vi "StdErr.vi"(11 "2D Array":u64[][](array[numeric]) format="%.1f") -> (0 "Deviation by row":i64[][](array[numeric]) format="%.1f", 1 "STD":dbl[](array[numeric]) format="%#_3g", 2 "Variance":dbl[](array[numeric]) format="%#_4g", 3 "Average by row":u64[](array[numeric]) format="%-2.1f", 4 "Mean as number":dbl format="%#_3g")   [LabVIEW 2023]
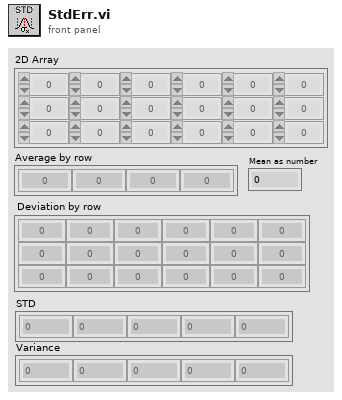
[diagram p1: front panel]
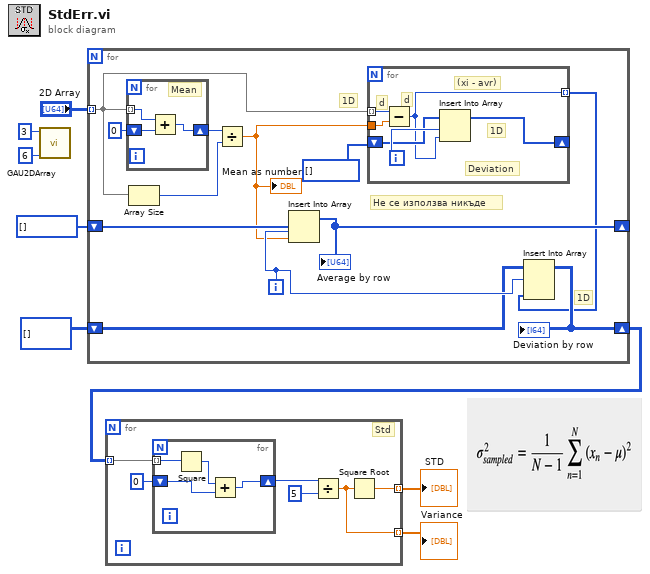
[diagram p0: block diagram]
diagram:
  n1 = call "GAU2DArray.vi"("Colums"=6, "Rows"=3) -> ()  [unwired: 8 in, 2 out]
  n2 = for {
    tunnel: "2D Array" -> [w11] mode=indexing
    shift-right: [w16] -> _
    shift-left: u64[] [] -> [w19]
    shift-right: [w13] -> w3
    shift-left: i64[][] [] -> [w14]
    i -> [w15]
    # "Не се използва никъде"
    # "1D"
    # "1D"
    n3 = for {
      tunnel: w11 -> [w29] mode=indexing
      shift-right: [w28] -> w18
      shift-left: 0 -> [w27]
      # "Mean"
      n4 = Add(x=w29, y=w27) -> (x+y=w28:u64)
    }
    n5 = Array Size(array=w11) -> (size(s)=w9:i32)
    n6 = Divide(x=w18, y=w9) -> (x/y=w12:dbl)
    "Mean as number" <- w12
    n7 = Insert Into Array(array=w19, index=w15, new element=w12) -> (w16:u64[])
    "Average by row" <- w16
    n8 = for {
      tunnel: w11 -> [w26] mode=indexing
      tunnel: w12 -> [w25]
      shift-right: [w22] -> _
      shift-left: u64[] [] -> [w23]
      tunnel: [w21] -> w10 mode=indexing
      i -> [w24]
      # "(xi - avr)"
      # "d"
      # "d"
      # "1D"
      # "Deviation"
      n9 = Subtract(x=w26, y=w25) -> (x-y=w21:i64)
      n10 = Insert Into Array "Insert Into Array"(array=w23, index=w24, new element=w21) -> (w22:u64[])
    }
    n11 = Insert Into Array "Insert Into Array"(array=w14, index (row)=w15, new element=w10) -> (w13:i64[][])  [unwired: 1 in]
    "Deviation by row" <- w13
  }
  n12 = for {
    tunnel: w3 -> [w35] mode=indexing
    tunnel: [w32] -> w2 mode=indexing
    tunnel: [w31] -> w1 mode=indexing
    # "Std"
    n13 = for {
      tunnel: w35 -> [w39] mode=indexing
      shift-right: [w37] -> w33
      shift-left: i64 0 -> [w36]
      n14 = Square(x=w39) -> (x^2=w38:i64)
      n15 = Add(x=w38, y=w36) -> (x+y=w37:i64)
    }
    n16 = Divide(x=w33, y=i64 5) -> (x/y=w31:dbl)
    n17 = Square Root(x=w31) -> (sqrt(x)=w32:dbl)
  }
  "STD" <- w2
  "Variance" <- w1
